vi "Angle_around_Z_axis.vi"(1 "gz":i32, 2 "dt":dbl=0.1 format="%#_13g") -> (0 "Angle around the Z-axis (*yaw)":dbl)   [LabVIEW 2015]
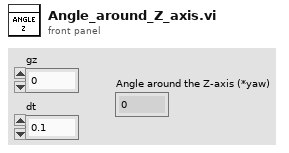
[diagram p1: front panel]
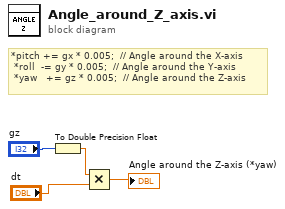
[diagram p0: block diagram]
diagram:
  # "*pitch += gx * 0.005;  // Angle around the X-axis\n *roll  -= gy * 0.005;  // Angle around the Y-axis\n *yaw   += gz * 0.005;  // Angle around the Z-axis"
  n1 = To Double Precision Float(number="gz") -> (double precision float=w1:dbl)
  n2 = Multiply(x=w1, y="dt") -> (x*y=→"Angle around the Z-axis (*yaw)":dbl)
